vi "queuePlay.vi"() -> ()   [LabVIEW 2011, in "run.lvlib"]
uses:
  run.lvlib
panel:
  out "Numeric":i32
  in  "stop":bool
  out "element":i32
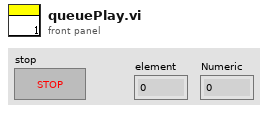
[diagram p1: front panel]
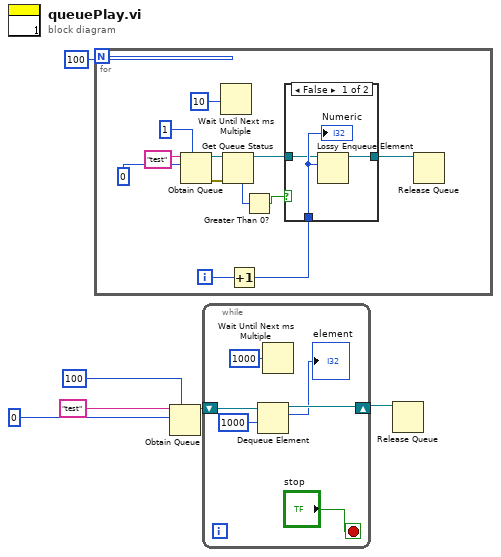
[diagram p0: block diagram]
diagram:
  n1 = for {
    N: 100 -> [_]
    i -> [w18]
    n2 = Obtain Queue(max queue size (-1, unlimited)=1, name (unnamed)="test", element data type=0) -> (queue out=w10:refnum<queue>, error out=w9:errorcluster)  [unwired: 2 in, 1 out]
    n3 = Wait Until Next ms Multiple(millisecond multiple=10) -> ()  [unwired: 1 out]
    n4 = Get Queue Status(queue=w10, error in (no error)=w9) -> (queue out=w17:refnum<queue>, # elements in queue=w16:i32)  [unwired: 1 in, 6 out]
    n5 = Increment(x=w18) -> (x+1=w14:i32)
    n6 = Greater Than 0?(x=w16) -> (x > 0?=w15:bool)
    n7 = case shown="False" w15 {
      tunnel: w14 -> [w21 _]
      tunnel: [w20 w22] -> w8
      tunnel: w17 -> [w19 w22]
      frame False {
        n8 = Lossy Enqueue Element(queue=w19, element=w21) -> (queue out=w20:refnum<queue>)  [unwired: 1 in, 3 out]
        "Numeric" <- w21
      }
      frame True {
      }
    }
    n9 = Release Queue(queue=w8) -> ()  [unwired: 2 in, 3 out]
  }
  n10 = Obtain Queue(max queue size (-1, unlimited)=100, name (unnamed)="test", element data type=0) -> (queue out=w2:refnum<queue>)  [unwired: 2 in, 2 out]
  n11 = while {
    shift-right: [w27] -> w1
    shift-left: w2 -> [w28]
    stop <- "stop" stop-if-true
    n12 = Dequeue Element(queue=w28, timeout in ms (-1)=1000) -> (queue out=w27:refnum<queue>, element=→"element":i32)  [unwired: 1 in, 2 out]
    n13 = Wait Until Next ms Multiple(millisecond multiple=1000) -> ()  [unwired: 1 out]
  }
  n14 = Release Queue(queue=w1) -> ()  [unwired: 2 in, 3 out]
